vi "AxXYGraph.vi"(2 "dx":dbl, 3 "N":dbl, 4 "x0":dbl) -> (0 "Multiplier":dbl, 1 "Offset":dbl)   [LabVIEW 2019]
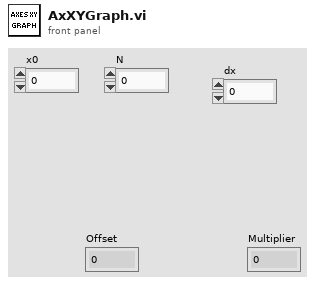
[diagram p1: front panel]
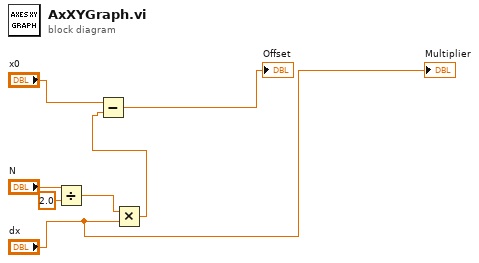
[diagram p0: block diagram]
diagram:
  n1 = Divide(x="N", y=2.0) -> (x/y=w4:dbl)
  n2 = Multiply(x=w4, y="dx") -> (x*y=w3:dbl)
  n3 = Subtract(x="x0", y=w3) -> (x-y=→"Offset":dbl)
  "Multiplier" <- "dx"
